vi "BetterJSON evaluation.vi"() -> ()   [LabVIEW 2017]
uses:
  Variant Tree.xctl
panel:
  out "Variant":variant
  in  "stop":bool
  in  "Variant Tree":variant(xcontrol)
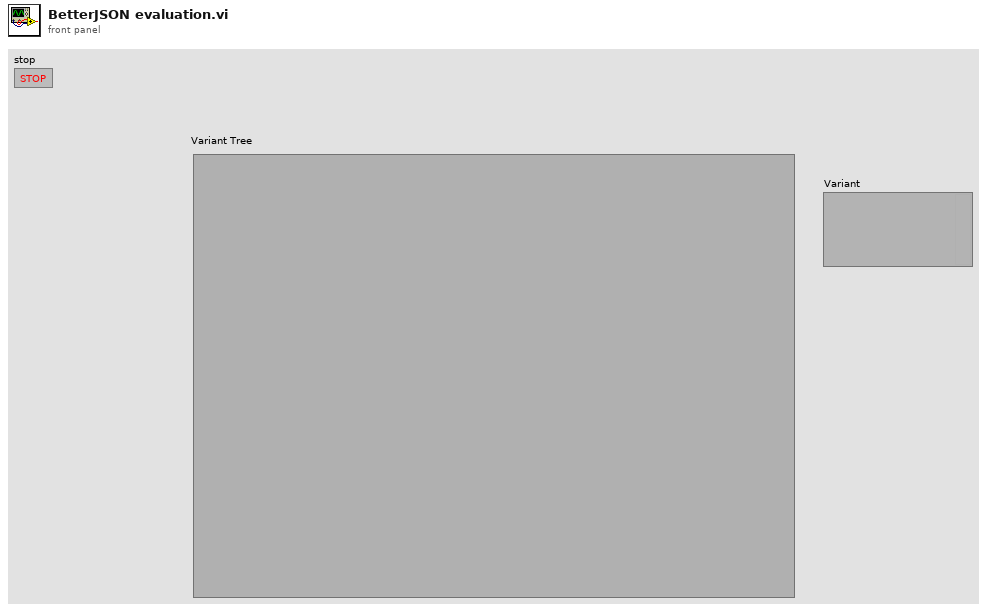
[diagram p1: front panel]
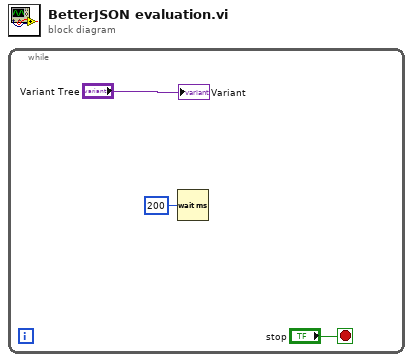
[diagram p0: block diagram]
diagram:
  n1 = while {
    stop <- "stop" stop-if-true
    n2 = Wait (ms)(milliseconds to wait=u32 200) -> ()  [unwired: 1 out]
    "Variant" <- "Variant Tree"
  }
